vi "rad_Deploy Application Image.vi"(7 "App Image Temp Folder":path=path "C:/dev/Architectures/Reference Designs/Application Deployment and Replication/Application Deployment Utility/trunk/source/Application Images/_temp", 8 "error in (no error)":errorcluster, 10 "Selected Targets":T1[](array[typedef]) {"Primary NIC"."IP Address Request Mode" items=["Static"=1, "DHCP/Link-Local"=2, "Link-Local Only"=4, "DHCP Only"=8]}, 11 "App Image Path":path=path "C:/dev/Architectures/Reference Designs/Application Deployment and Replication/Application Deployment Utility/trunk/source/Application Images/AppImage1.lvappimg") -> (0 "error out":errorcluster, 1 "Cancelled":bool)   [LabVIEW 2021]
uses:
  Targets/TypeDefs/rad_Target Information.ctl
  Targets/TypeDefs/rad_Target Network Settings.ctl
  TypeDefs/rad_Target Configuration Settings.ctl
  TypeDefs/rad_Target Configuration Operations.ctl
  TypeDefs/rad_Deployment Notifiers.ctl
  TypeDefs/rad_Deployment Status Data Type.ctl
  TypeDefs/rad_Deployment Progress Data Type.ctl
  Util/FP Control/FP Control Functions.ctl
  <vilib>/Utility/error.llb/Clear Errors.vi
  NI-Auth/rad_IPaddr and Password Global.vi
  rad_Globals.vi
  <vilib>/nisyscfg/Initialize Session.vi
  <vilib>/nisyscfg/Close (System).vi
  NI-Auth/rad_Open Session.vi
  <vilib>/nisyscfg/nisyscfg.lvlib
panel:
  out "Stop Updates":bool
  in  "Deploy":bool
  in  "Config Options":bool
  in  "Log":bool
  in  "Stop":bool
  in  "State Variables":T6={"App Image Path"=path "C:/dev/Architectures/Reference Designs/Application Deployment and Replication/Application Deployment Utility/trunk/source/Application Images/AppImage1.lvappimg", "App Image Temp Folder"=path "C:/dev/Architectures/Reference Designs/Application Deployment and Replication/Application Deployment Utility/trunk/source/Application Images/_temp", "Targets"=[], "Target Configuration Options"={"NumInBatch"=0, "Target Config Operation"=enum."No Config", "Target Name"="", "Increment Static IPs"=FALSE, "Change Target Name"=FALSE, "Primary NIC"={"MAC address"="", "IP Address Request Mode"=2, "IP address"="", "Subnet mask"="", "Gateway"="", "DNS server"=""}}, "Deployment Notifiers"=[]} {"Target Configuration Options"."Primary NIC"."IP Address Request Mode" items=["Static"=1, "DHCP/Link-Local"=2, "Link-Local Only"=4, "DHCP Only"=8]; "Targets"."Primary NIC"."IP Address Request Mode" items=["Static"=1, "DHCP/Link-Local"=2, "Link-Local Only"=4, "DHCP Only"=8]}
  out "Targets":i32(listbox)
  in  "Close":bool
  # "Targets"
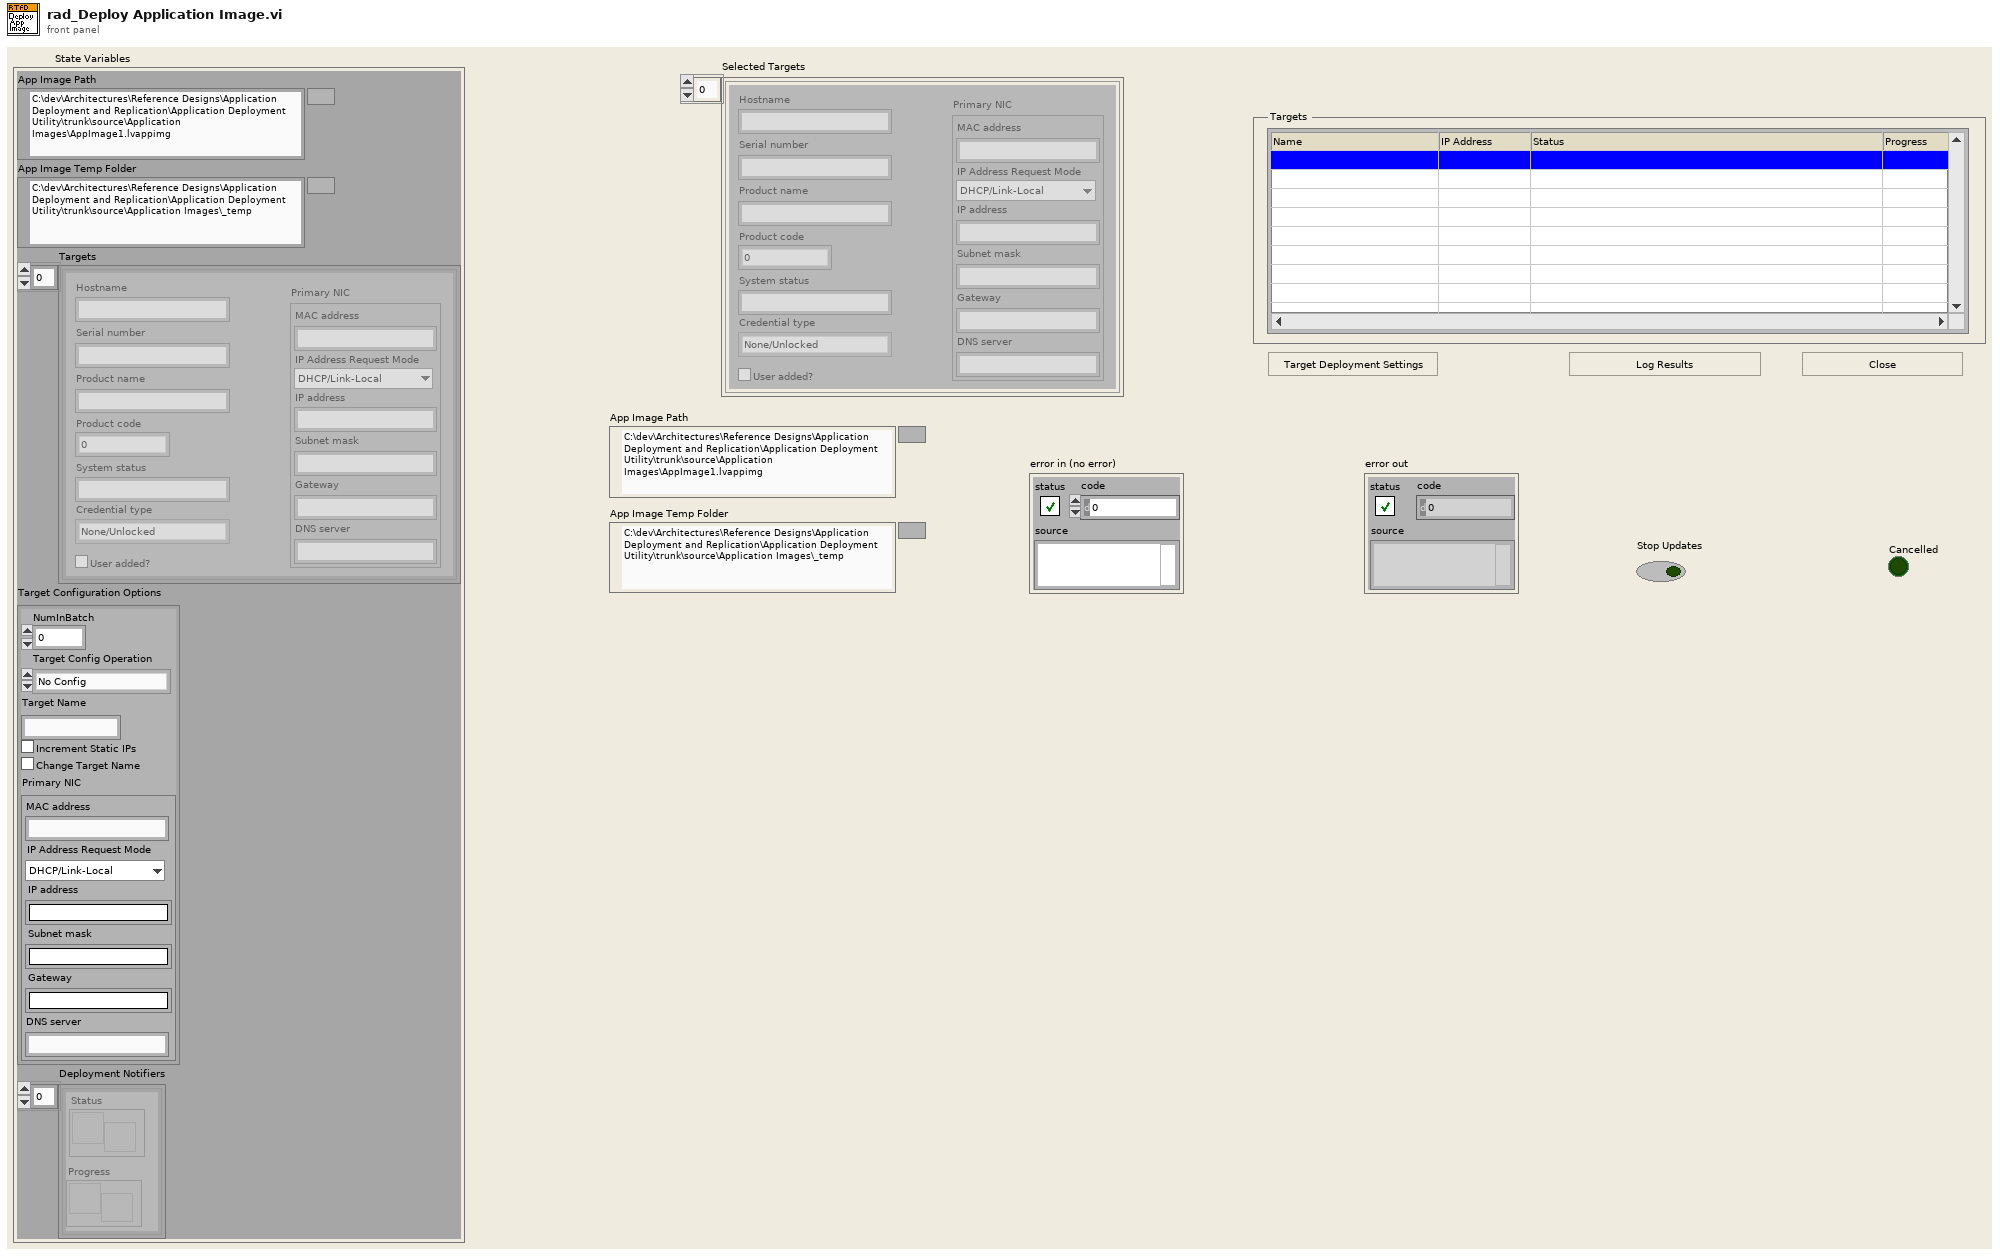
[diagram p1: front panel]
types:
  T1 = typedef "rad_Target Information.ctl" = cluster{"Hostname":string, "Serial number":string, "Product name":string, "Product code":i32, "System status":string, "Credential type":enum16{"None/Unlocked", "FTP Password", "NIAuth Credentials"}, "User added?":bool, "Primary NIC":T2}
  T2 = typedef "rad_Target Network Settings.ctl" = cluster{"MAC address":string, "IP Address Request Mode":i32, "IP address":string, "Subnet mask":string, "Gateway":string, "DNS server":string}
  T3 = typedef "rad_Target Configuration Settings.ctl" = cluster{"NumInBatch":u32, "Target Config Operation":T4, "Target Name":string, "Increment Static IPs":bool, "Change Target Name":bool, "Primary NIC":T2}
  T4 = typedef "rad_Target Configuration Operations.ctl" = enum8{"No Config", "Image Config", "Static Config"}
  T5 = typedef "rad_Deployment Notifiers.ctl" = cluster{"Status":refnum<notifier>, "Progress":refnum<notifier>}
  T6 = cluster{"App Image Path":path, "App Image Temp Folder":path, "Targets":T1[], "Target Configuration Options":T3, "Deployment Notifiers":T5[]}
  T7 = typedef "rad_Deployment Progress Data Type.ctl" = i8
  T8 = typedef "rad_Deployment Status Data Type.ctl" = string
  T9 = typedef "FP Control Functions.ctl" = enum16{"Open", "Close", "Bring To Front", "Center"}
  T10 = enum8{"Enabled", "Disabled", "Disabled and Grayed Out"}
  T11 = typedef "rad_Application Image Properties.ctl" = cluster{"Name":string, "Version":string, "Time":timestamp, "Description":string, "Key":string, "Chassis":string, "FPGA Properties":T12, "Model":string, "Retrieve":string[], "Deploy":string[], "Installed Software":string[]}
  T12 = typedef "rad_FPGA Properties.ctl" = T13[]
  T13 = typedef "rad_FPGA Flash Properties.ctl" = cluster{"Resource Name":string, "Path":path}
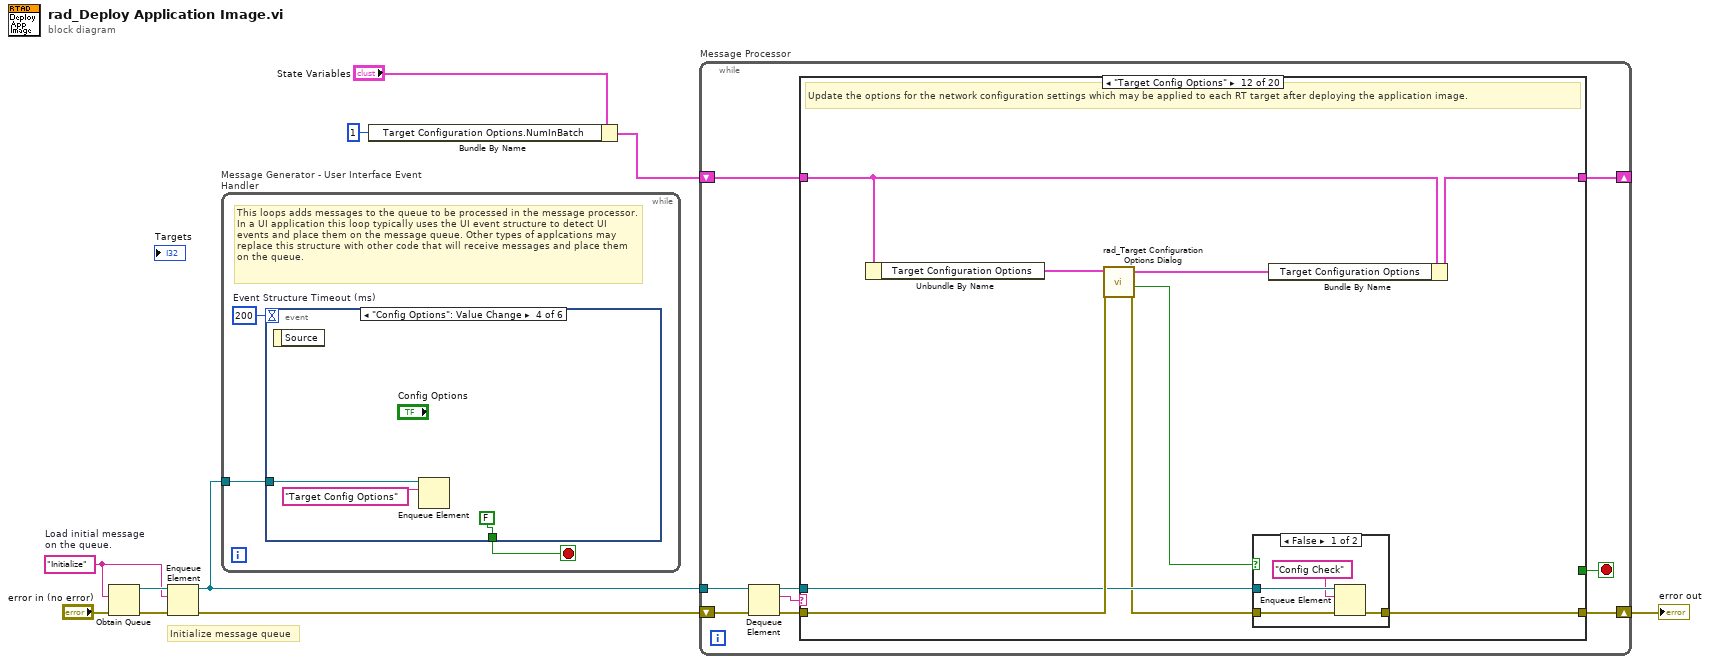
[diagram p0: block diagram]
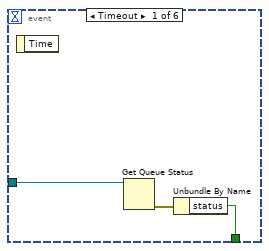
[diagram p2: hidden frame]
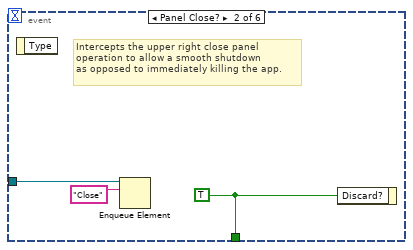
[diagram p3: hidden frame]
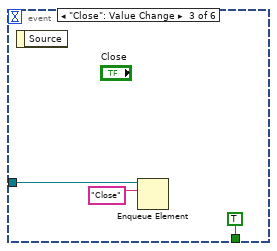
[diagram p4: hidden frame]
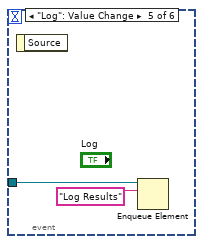
[diagram p5: hidden frame]
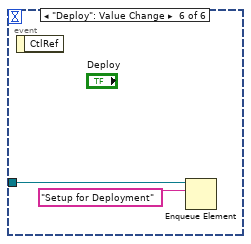
[diagram p6: hidden frame]
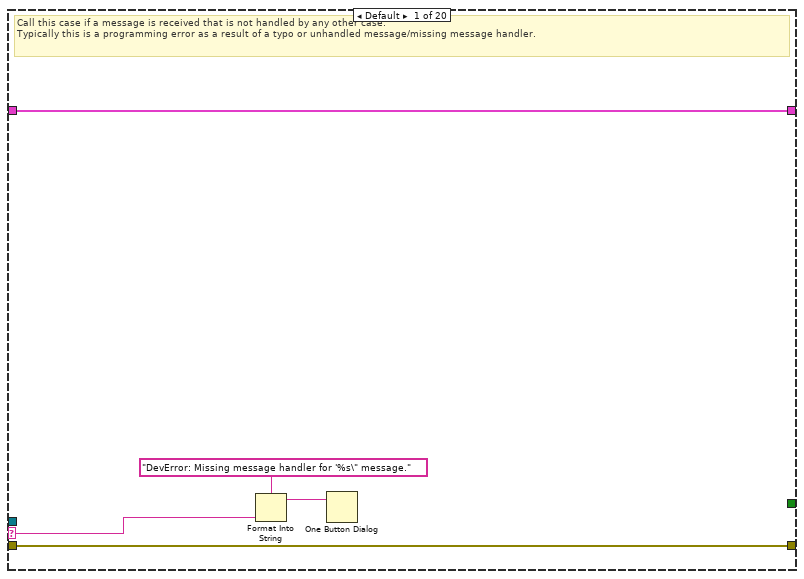
[diagram p7: hidden frame]
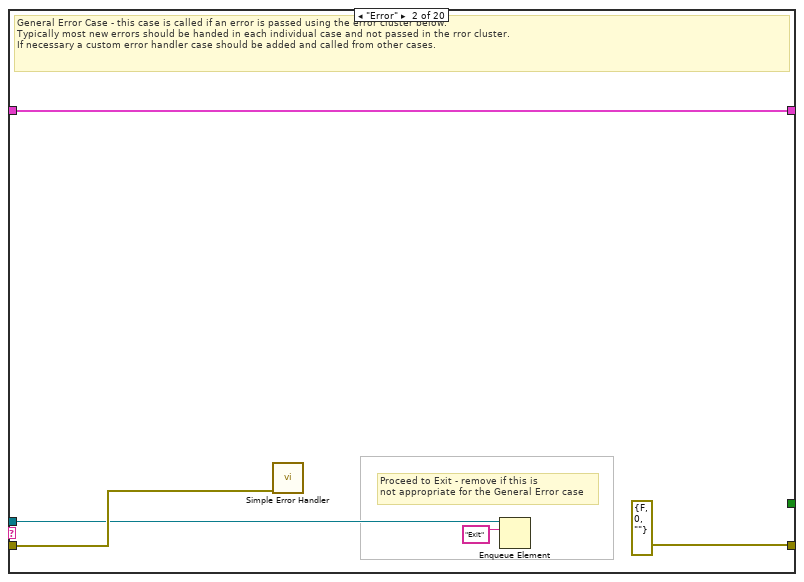
[diagram p8: hidden frame]
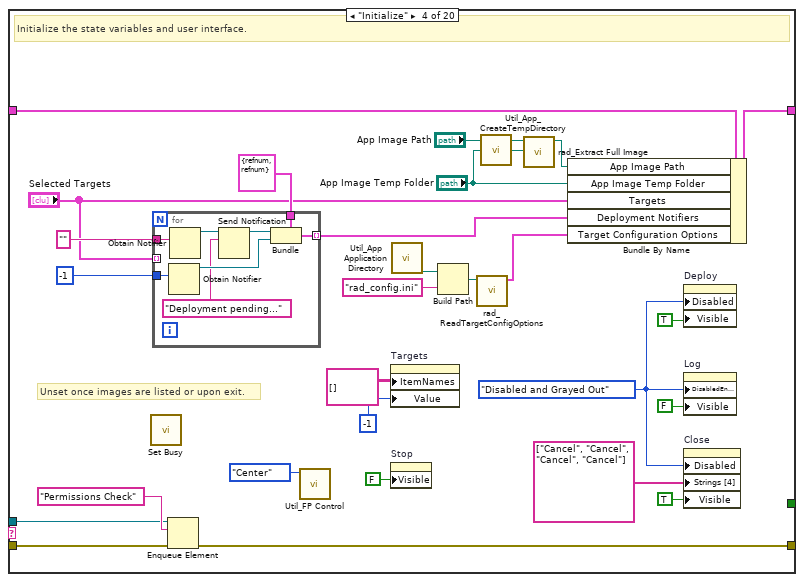
[diagram p10: hidden frame]
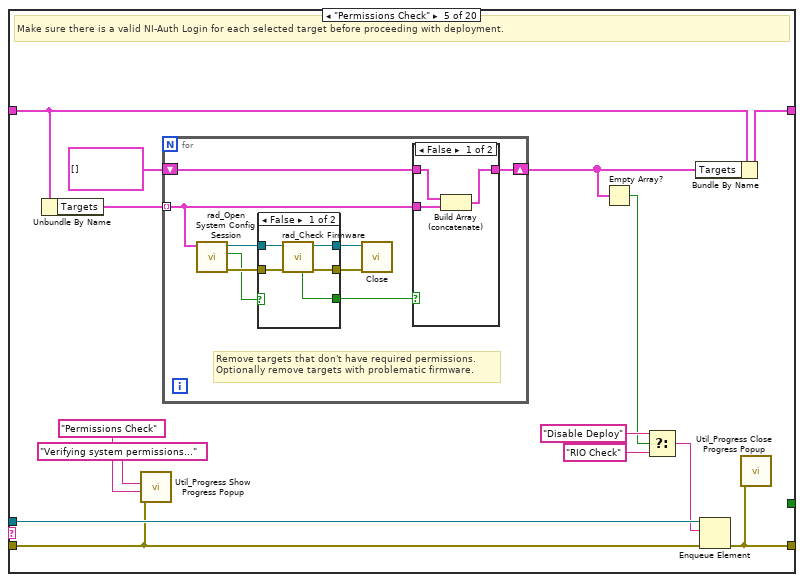
[diagram p11: hidden frame]
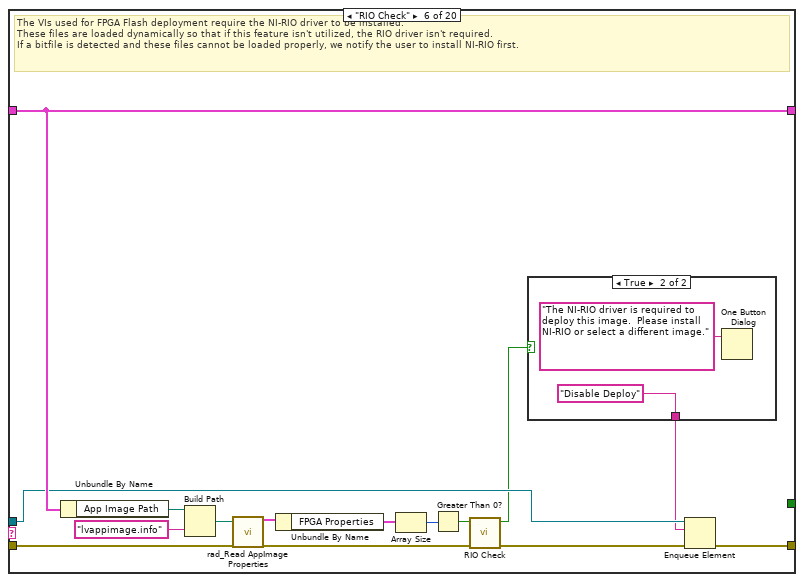
[diagram p14: hidden frame]
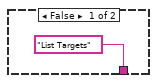
[diagram p15: hidden frame]
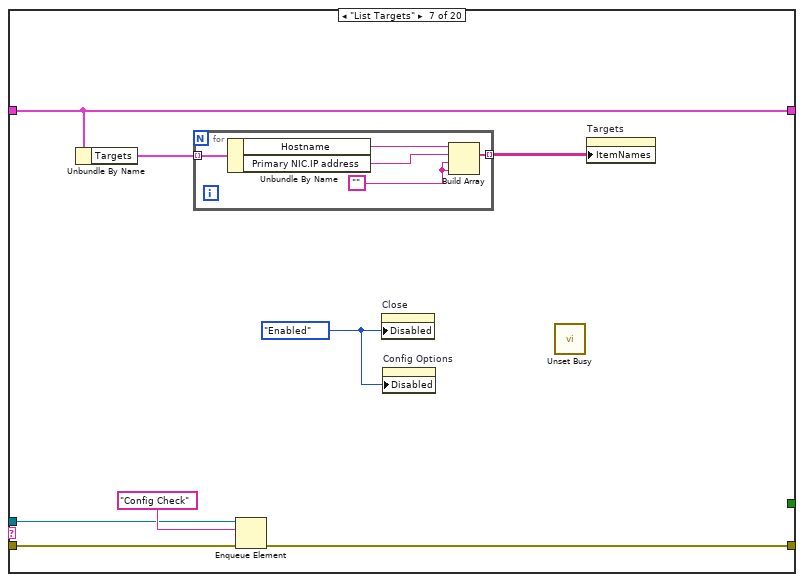
[diagram p16: hidden frame]
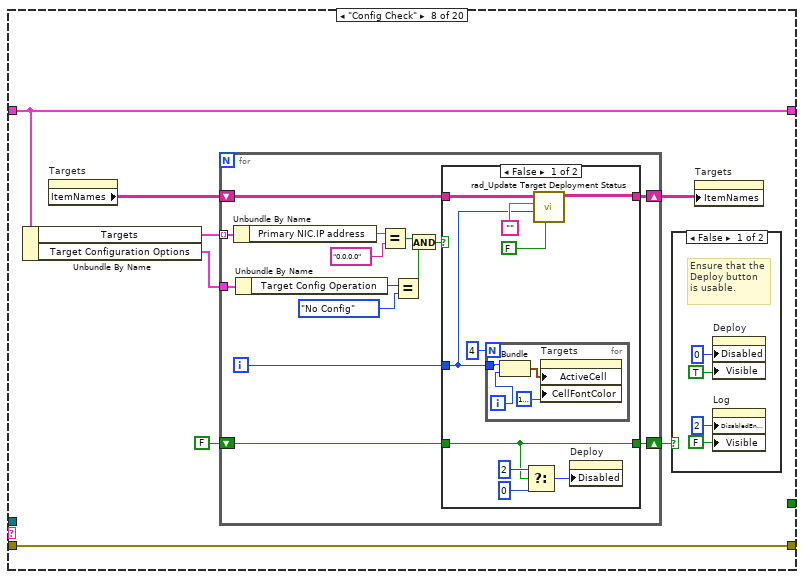
[diagram p17: hidden frame]
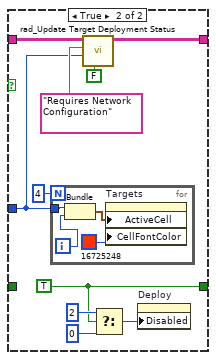
[diagram p19: hidden frame]
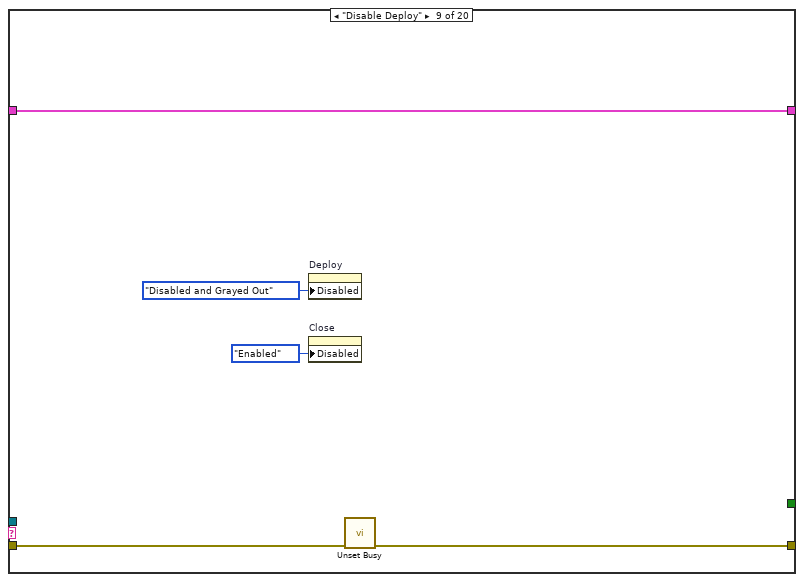
[diagram p20: hidden frame]
diagram:
  w4 = "Initialize"  # Load initial message on the queue.
  # "Initialize message queue"
  n1 = Obtain Queue(element data type=w4, error in (no error)="error in (no error)") -> (queue out=w6:refnum<queue>, error out=w10:errorcluster)  [unwired: 3 in, 1 out]
  n2 = Enqueue Element(queue=w6, element=w4, error in (no error)=w10) -> (queue out=w5:refnum<queue>, error out=w7:errorcluster)  [unwired: 1 in, 1 out]
  n3 = while "Message Generator - User Interface Event Handler" {
    tunnel: w5 -> [w11]
    stop <- w12 stop-if-true
    w13 = 200  # Event Structure Timeout (ms)
    # "This loops adds messages to the queue to be processed in the message processor. In a UI application this loop typically uses the UI event structure to detect UI events and place them on the message queue. Other types of applcations may replace this structure with other code that will receive messages and place them on the queue."
    n4 = event shown="[3] \"Config Options\": Value Change" {
      selector: _ -> [_ _ _ _ _ _]
      dyn-events: _ -> [_ _ _ _ _ _]
      timeout: w13 -> [_ _ _ _ _ _]
      tunnel: [w15 w19 TRUE ("Discard?") FALSE ("Discard?") _ _] -> w12
      tunnel: w11 -> [w14 w18 w22 w25 w27 w29]
      event Timeout {
        n5 = event-data() -> ()  [unwired: 2 out]
        n6 = Get Queue Status(queue=w14) -> (error out=w16:errorcluster)  [unwired: 2 in, 7 out]
        n7 = Unbundle By Name(w16) -> ("status"=w15:bool)
      }
      event Panel Close? {
        w19 = TRUE ("Discard?")
        # "Intercepts the upper right close panel\noperation to allow a smooth shutdown\nas opposed to immediately killing the app."
        n8 = event-data() -> ()  [unwired: 2 out]
        n9 = Enqueue Element(queue=w18, element="Close") -> ()  [unwired: 2 in, 3 out]
        n10 = event-data("Discard?"=w19) -> ()  [unwired: 1 in, 1 out]
      }
      event "Close": Value Change {
        n11 = event-data() -> ()  [unwired: 2 out]
        n12 = Enqueue Element(queue=w22, element="Close") -> ()  [unwired: 2 in, 3 out]
      }
      event "Config Options": Value Change {
        n13 = event-data() -> ()  [unwired: 2 out]
        n14 = Enqueue Element(queue=w25, element="Target Config Options") -> ()  [unwired: 2 in, 3 out]
      }
      event "Log": Value Change {
        n15 = event-data() -> ()  [unwired: 2 out]
        n16 = Enqueue Element(queue=w27, element="Log Results") -> ()  [unwired: 2 in, 3 out]
      }
      event "Deploy": Value Change {
        n17 = event-data() -> ()  [unwired: 2 out]
        n18 = Enqueue Element(queue=w29, element="Setup for Deployment") -> ()  [unwired: 2 in, 3 out]
      }
    }
  }
  n19 = Bundle By Name(cluster="State Variables", "Target Configuration Options.NumInBatch"=u32 1) -> (w2:T6)
  n20 = while "Message Processor" {
    shift-left: w7 -> [w33]
    shift-right: [w34] -> w8
    tunnel: w5 -> [w32]
    shift-left: w2 -> [w38]
    shift-right: [w37] -> _
    stop <- w30 stop-if-true
    n21 = Dequeue Element(queue=w32, error in (no error)=w33) -> (queue out=w36:refnum<queue>, element=w31:string, error out=w35:errorcluster)  [unwired: 1 in, 1 out]
    n22 = case shown="\"Target Config Options\"" w31 {
      selector: w31 -> [w41 _ _ _ _ _ _ _ _ _ _ _ _ _ _ _ _ _ _ _]
      tunnel: [w43 w48 w50 w77 w97 w133 w145 w155 w209 w213 w215 w221 w241 w260 w297 w305 w307 w315 w318 w325] -> w37
      tunnel: w38 -> [w43 w48 w50 w78 w98 w133 w145 w155 w209 w213 w215 w222 w241 w260 w297 w305 w307 w315 w318 w325]
      tunnel: w36 -> [_ w45 _ w56 w96 w130 w140 _ _ _ _ w219 w237 w255 _ _ _ w309 _ w330]
      tunnel: w35 -> [w42 w46 w49 w72 w92 w125 w142 w160 w211 w212 w214 w223 w242 w259 w298 w303 w306 w310 w316 w331]
      tunnel: [w42 errorcluster {"status"=FALSE, "code"=0, "source"=""} ("error out") w49 w58 w91 w131 w141 w160 w210 w212 w214 w217 w233 w253 w298 w302 w306 w308 w316 w322] -> w34
      tunnel: [_ _ _ _ _ _ _ _ _ _ _ _ _ _ _ _ _ _ _ TRUE] -> w30
      frame Default {
        # "Call this case if a message is received that is not handled by any other case.\nTypically this is a programming error as a result of a typo or unhandled message/missing message handler."
        n23 = Format Into String(format string="DevError: Missing message handler for '%s\" message." ("message"), w41) -> (resulting string=w39:string)  [unwired: 2 in, 1 out]
        n24 = One Button Dialog(message=w39) -> ()  [unwired: 2 out]
      }
      frame "Error" {
        # "Proceed to Exit - remove if this is\nnot appropriate for the General Error case"
        # "General Error Case - this case is called if an error is passed using the error cluster below.\nTypically most new errors should be handed in each individual case and not passed in the rror cluster.\nIf necessary a custom error handler case should be added and called from other cases."
        n25 = call <vilib>:"Simple Error Handler.vi"("error in (no error)"=w46) -> ()  [unwired: 1 in, 8 out]
        n26 = Enqueue Element(queue=w45, element="Exit") -> ()  [unwired: 2 in, 3 out]
      }
      frame "*******Init******" {
        # "Dummy case to add a seperator in the Case Structure menu."
      }
      frame "Initialize" {
        w51 = T10."Disabled and Grayed Out" ("Disabled")
        # "Unset once images are listed or upon exit."
        # "Initialize the state variables and user interface."
        n27 = call <vilib>:"Set Busy.vi"() -> ()  [unwired: 10 in, 2 out]
        n28 = for {
          tunnel: T8 "" ("status notifier data type") -> [w86]
          tunnel: T7 -1 ("Progress") -> [w85]
          tunnel: T5 {"Status"=refnum, "Progress"=refnum} ("Deployment Notifiers") -> [w83]
          tunnel: [w82] -> w67 mode=indexing
          tunnel: "Selected Targets" -> [_] mode=indexing
          n29 = Obtain Notifier(notification data type=w85) -> (notifier out=w84:refnum<notifier>)  [unwired: 3 in, 2 out]
          n30 = Obtain Notifier(notification data type=w86) -> (notifier out=w81:refnum<notifier>)  [unwired: 3 in, 2 out]
          n31 = Send Notification(notification=T8 "Deployment pending...", notifier=w81) -> (notifier out=w80:refnum<notifier>)  [unwired: 1 in, 1 out]
          n32 = Bundle(cluster=w83, "Status"=w80, "Progress"=w84) -> (w82:T5)
        }
        n33 = Enqueue Element(queue=w56, element="Permissions Check", error in (no error)=w72) -> (error out=w58:errorcluster)  [unwired: 1 in, 2 out]
        n34 = call "Util_FP Control.vi"("Function"=FP_Control_Functions."Center") -> ()  [unwired: 1 in, 10 out]
        n35 = property on="Targets" class="MCListbox (strict)"("ItemNames"=string[][] [] ("Item Names"), "Value"=-1 ("Targets")) -> ()  [unwired: 2 in, 2 out]
        n36 = property on="Stop" class="Bool"("Visible"=FALSE) -> ()  [unwired: 2 in, 2 out]
        n37 = call "Util_App Application Directory.vi"() -> ("Application Directory"=w66:path)  [unwired: 11 out]
        n38 = Build Path(base path=w66, name or relative path="rad_config.ini" ("Config File Name")) -> (appended path=w64:path)
        n39 = call "rad_ReadTargetConfigOptions.vi"("configuration file path"=w64) -> ("TargetConfigurationOptions"=w63:T3)  [unwired: 9 in, 1 out]
        n40 = call "Util_App_CreateTempDirectory.vi"("TempFolderPath"="App Image Temp Folder") -> ("TempFolderPath_out"=w60:path)
        n41 = call "rad_Extract Full Image.vi"("App Image Temp Folder"=w60, "Zipped App Image File Path"="App Image Path") -> ("Unzipped App Image Folder Path"=w61:path)  [unwired: 8 in, 1 out]
        n42 = Bundle By Name(cluster=w78, "App Image Path"=w61, "App Image Temp Folder"="App Image Temp Folder", "Targets"="Selected Targets", "Deployment Notifiers"=w67, "Target Configuration Options"=w63) -> (w77:T6)
        n43 = property on="Deploy" class="Bool"("Disabled"=w51, "Visible"=TRUE) -> ()  [unwired: 2 in, 2 out]
        n44 = property on="Log" class="Bool"("DisabledEnum"=w51, "Visible"=FALSE) -> ()  [unwired: 2 in, 2 out]
        n45 = property on="Close" class="Bool"("Disabled"=w51, "Strings [4]"=string[] ["Cancel", "Cancel", "Cancel", "Cancel"], "Visible"=TRUE) -> ()  [unwired: 2 in, 2 out]
      }
      frame "Permissions Check" {
        # "Make sure there is a valid NI-Auth Login for each selected target before proceeding with deployment."
        n46 = Unbundle By Name(w98) -> ("Targets"=w100:T1[])
        n47 = call "Util_Progress Show Progress Popup.vi"("error in (no error)"=w92, "Title"="Permissions Check" ("Message"), "Message"="Verifying system permissions...") -> ()  [unwired: 8 in, 1 out]
        n48 = for {
          tunnel: w100 -> [w107] mode=indexing
          shift-right: [w109] -> w88
          shift-left: T1[] [] -> [w108]
          # "Remove targets that don't have required permissions.\nOptionally remove targets with problematic firmware."
          n49 = call "rad_Open System Config Session.vi"("Target settings"=w107) -> ("error out"=w106:errorcluster, "Cancelled"=w101:bool, "Session out"=w104:refnum<k21>)  [unwired: 7 in, 1 out]
          n50 = case shown="False" w101 {
            selector: w101 -> [_ w115]
            tunnel: w106 -> [w114 w117]
            tunnel: [w111 w117] -> w105
            tunnel: w104 -> [w113 w116]
            tunnel: [w112 w116] -> w103
            tunnel: [w110 w115] -> w102
            frame False {
              n51 = call "rad_Check Firmware.vi"("error in (no error)"=w114, "System Configuration"=w113) -> ("error out"=w111:errorcluster, "System Configuration out"=w112:refnum<k21>, "Bad firmware and user canceled"=w110:bool)  [unwired: 7 in]
            }
            frame True {
            }
          }
          n52 = call-poly <vilib>:"Close.vi"("error in (no error)"=w105, "Session in"=w103) -> ()  [unwired: 9 in, 1 out]
          n53 = case shown="False" w102 {
            tunnel: w107 -> [w120 _]
            tunnel: [w119 w121] -> w109
            tunnel: w108 -> [w118 w121]
            frame False {
              n54 = Build Array (concatenate)(w118, w120) -> (w119:T1[])
            }
            frame True {
            }
          }
        }
        n55 = Empty Array?(array=w88) -> (empty?=w87:bool)
        n56 = Select(t="Disable Deploy", s=w87, f="RIO Check") -> (s? t:f=w93:string)
        n57 = Bundle By Name(cluster=w98, "Targets"=w88) -> (w97:T6)
        n58 = Enqueue Element(queue=w96, element=w93, error in (no error)=w92) -> (error out=w91:errorcluster)  [unwired: 1 in, 2 out]
        n59 = call "Util_Progress Close Progress Popup.vi"("error in (no error)"=w91) -> ()  [unwired: 10 in, 1 out]
      }
      frame "RIO Check" {
        # "The VIs used for FPGA Flash deployment require the NI-RIO driver to be installed.  \nThese files are loaded dynamically so that if this feature isn't utilized, the RIO driver isn't required.\nIf a bitfile is detected and these files cannot be loaded properly, we notify the user to install NI-RIO first."
        n60 = Unbundle By Name(w133) -> ("App Image Path"=w123:path)
        n61 = Build Path(base path=w123, name or relative path="lvappimage.info") -> (appended path=w122:path)
        n62 = call "rad_Read AppImage Properties.vi"("AppImage Properties Path"=w122, "error in (no error)"=w125) -> ("AppImage Properties"=w126:T11, "error out"=w127:errorcluster)  [unwired: 12 in, 4 out]
        n63 = Unbundle By Name(w126) -> ("FPGA Properties"=w136:T12)
        n64 = Array Size(array=w136) -> (size(s)=w135:i32)
        n65 = Greater Than 0?(x=w135) -> (x > 0?=w134:bool)
        n66 = call "RIO Check.vi"("error in"=w127, "Requires RIO"=w134) -> ("error out"=w132:errorcluster, "RIO needed but not installed"=w129:bool)  [unwired: 8 in]
        n67 = case shown="True" w129 {
          tunnel: ["List Targets" "Disable Deploy" ("t")] -> w128
          frame False {
          }
          frame True {
            n68 = One Button Dialog(message="The NI-RIO driver is required to deploy this image.  Please install NI-RIO or select a different image.") -> ()  [unwired: 1 in, 1 out]
          }
        }
        n69 = Enqueue Element(queue=w130, element=w128, error in (no error)=w132) -> (error out=w131:errorcluster)  [unwired: 1 in, 2 out]
      }
      frame "List Targets" {
        w144 = T10."Enabled" ("Disabled")
        n70 = Unbundle By Name(w145) -> ("Targets"=w147:T1[])
        n71 = for {
          tunnel: w147 -> [w152] mode=indexing
          tunnel: [w149] -> w146 mode=indexing
          w148 = ""
          n72 = Unbundle By Name(w152) -> ("Hostname"=w151:string, "Primary NIC.IP address"=w150:string)
          n73 = Build Array(w151, w150, w148, w148) -> (w149:string[])
        }
        n74 = Enqueue Element(queue=w140, element="Config Check", error in (no error)=w142) -> (error out=w141:errorcluster)  [unwired: 1 in, 2 out]
        n75 = property on="Close" class="Bool"("Disabled"=w144) -> ()  [unwired: 2 in, 2 out]
        n76 = property on="Config Options" class="Bool"("Disabled"=w144) -> ()  [unwired: 2 in, 2 out]
        n77 = call <vilib>:"Unset Busy.vi"() -> ()  [unwired: 11 in, 1 out]
        n78 = property on="Targets" class="MCListbox (strict)"("ItemNames"=w146) -> ()  [unwired: 2 in, 2 out]
      }
      frame "Config Check" {
        n79 = Unbundle By Name(w155) -> ("Targets"=w158:T1[], "Target Configuration Options"=w159:T3)
        n80 = property on="Targets" class="MCListbox (strict)"() -> ("ItemNames"=w154:string[][])  [unwired: 2 in, 2 out]
        n81 = for {
          tunnel: w158 -> [w169] mode=indexing
          tunnel: w159 -> [w168]
          shift-right: [w165] -> w153
          shift-left: FALSE -> [w166]
          shift-right: [w171] -> w156
          shift-left: w154 -> [w167]
          i -> [w170]
          n82 = Unbundle By Name(w169) -> ("Primary NIC.IP address"=w178:string)
          n83 = Unbundle By Name(w168) -> ("Target Config Operation"=w176:T4)
          n84 = Equal?(x=w178, y="0.0.0.0") -> (x = y?=w174:bool)
          n85 = Equal?(x=w176, y=rad_Target_Configuration_Operations."No Config") -> (x = y?=w172:bool)
          n86 = And(x=w174, y=w172) -> (x .and. y?=w173:bool)
          n87 = case shown="False" w173 {
            tunnel: [w187 w202] -> w171
            tunnel: w170 -> [w185 w198]
            tunnel: w167 -> [w188 w199]
            tunnel: w166 -> [w180 _]
            tunnel: [w180 w195] -> w165
            frame False {
              n88 = for {
                N: 4 -> [_]
                tunnel: w185 -> [w191]
                i -> [w190]
                n89 = Bundle(w191, w190) -> (w189:cluster{i32, i32})  [unwired: 1 in]
                n90 = property on="Targets" class="MCListbox (strict)"("ActiveCell"=w189, "CellFontColor"=u32 16777222) -> ()  [unwired: 2 in, 2 out]
              }
              n91 = Select(t=2, s=w180, f=0) -> (s? t:f=w181:i32)
              n92 = call "rad_Update Target Deployment Status.vi"("Add Timestamp?"=FALSE, "Target Index"=w185, "Message"="", "Targets Deployment Status"=w188) -> ("Targets Deployment Status"=w187:string[][])  [unwired: 7 in]
              n93 = property on="Deploy" class="Bool"("Disabled"=w181) -> ()  [unwired: 2 in, 2 out]
            }
            frame True {
              w195 = TRUE
              n94 = for {
                N: 4 -> [_]
                tunnel: w198 -> [w205]
                i -> [w204]
                n95 = Bundle(w205, w204) -> (w203:cluster{i32, i32})  [unwired: 1 in]
                n96 = property on="Targets" class="MCListbox (strict)"("ActiveCell"=w203, "CellFontColor"=u32 16725248) -> ()  [unwired: 2 in, 2 out]
              }
              n97 = call "rad_Update Target Deployment Status.vi"("Add Timestamp?"=FALSE, "Target Index"=w198, "Message"="Requires Network Configuration", "Targets Deployment Status"=w199) -> ("Targets Deployment Status"=w202:string[][])  [unwired: 7 in]
              n98 = Select(t=2, s=w195, f=0) -> (s? t:f=w194:i32)
              n99 = property on="Deploy" class="Bool"("Disabled"=w194) -> ()  [unwired: 2 in, 2 out]
            }
          }
        }
        n100 = case shown="False" w153 {
          frame False {
            # "Ensure that the\nDeploy button\nis usable."
            n101 = property on="Deploy" class="Bool"("Disabled"=0, "Visible"=TRUE) -> ()  [unwired: 2 in, 2 out]
            n102 = property on="Log" class="Bool"("DisabledEnum"=2, "Visible"=FALSE) -> ()  [unwired: 2 in, 2 out]
          }
          frame True {
          }
        }
        n103 = property on="Targets" class="MCListbox (strict)"("ItemNames"=w156) -> ()  [unwired: 2 in, 2 out]
      }
      frame "Disable Deploy" {
        n104 = property on="Deploy" class="Bool"("Disabled"=T10."Disabled and Grayed Out") -> ()  [unwired: 2 in, 2 out]
        n105 = property on="Close" class="Bool"("Disabled"=T10."Enabled") -> ()  [unwired: 2 in, 2 out]
        n106 = call <vilib>:"Unset Busy.vi"("error in (no error)"=w211) -> ("error out"=w210:errorcluster)  [unwired: 10 in]
      }
      frame "*****************" {
        # "Dummy case to add a seperator in the Case Structure menu."
      }
      frame "Update Display" {
      }
      frame "Target Config Options" {
        # "Update the options for the network configuration settings which may be applied to each RT target after deploying the application image."
        n107 = Unbundle By Name(w222) -> ("Target Configuration Options"=w224:T3)
        n108 = call "rad_Target Configuration Options Dialog.vi"("error in"=w223, "Target Configuration Options"=w224) -> ("error out"=w218:errorcluster, "Cancelled"=w216:bool, "Target Configuration Options"=w220:T3)  [unwired: 7 in]
        n109 = case shown="False" w216 {
          tunnel: w219 -> [w228 _]
          tunnel: w218 -> [w227 w229]
          tunnel: [w226 w229] -> w217
          frame False {
            n110 = Enqueue Element(queue=w228, element="Config Check" ("Message Name"), error in (no error)=w227) -> (error out=w226:errorcluster)  [unwired: 1 in, 2 out]
          }
          frame True {
          }
        }
        n111 = Bundle By Name(cluster=w222, "Target Configuration Options"=w220) -> (w221:T6)
      }
      frame "Setup for Deployment" {
        w239 = T10."Disabled and Grayed Out" ("Disabled")
        # "Update the UI for the deployment process - disable some buttons."
        n112 = Enqueue Element(queue=w237, element="Deploy Application Image", error in (no error)=w242) -> (queue out=w234:refnum<queue>, error out=w235:errorcluster)  [unwired: 1 in, 1 out]
        n113 = property on="Stop" class="Bool"("Visible"=TRUE) -> ()  [unwired: 2 in, 2 out]
        n114 = property on="Close" class="Bool"("Disabled"=w239, "Visible"=FALSE) -> ()  [unwired: 2 in, 2 out]
        n115 = property on="Config Options" class="Bool"("Disabled"=w239) -> ()  [unwired: 2 in, 2 out]
        n116 = property on="Log" class="Bool"("Disabled"=w239, "Visible"=TRUE) -> ()  [unwired: 2 in, 2 out]
        n117 = Enqueue Element(queue=w234, element="Cleanup from Deployment", error in (no error)=w235) -> (error out=w233:errorcluster)  [unwired: 1 in, 2 out]
        n118 = property on="Deploy" class="Bool"("Visible"=FALSE) -> ()  [unwired: 2 in, 2 out]
      }
      frame "Deploy Application Image" {
        # "Deploy the specified image to the selected targets in parallel, in batches up to the Deployment Batch Size.\nIf an error occurs, display it for the relevant target, but don't pass it out the error wire.\nThis allows deployment to succeed for as many targets as possible."
        n119 = Unbundle By Name(w260) -> ("Deployment Notifiers"=w250:T5[], "App Image Temp Folder"=w261:path, "App Image Path"=w263:path, "Targets"=w262:T1[], "Target Configuration Options"=w244:T3)
        n120 = control-ref of="Targets"() -> (w251:refnum<vi>)
        n121 = control-ref of="Stop Updates"() -> (w246:refnum<vi>)
        n122 = Unbundle By Name(w244) -> ("NumInBatch"=w243:u32)
        n123 = Array Size(array=w250) -> (size(s)=w258:i32)
        n124 = Divide(x=w258, y=w243) -> (x/y=w257:dbl)
        n125 = Round Toward +Infinity(x=w257) -> (ceil(x): smallest int >= x=w256:dbl)
        n126 = for {
          N: w256 -> [_]
          tunnel: w263 -> [w290]
          tunnel: w262 -> [w285]
          tunnel: w261 -> [w289]
          tunnel: w243 -> [w282]
          shift-right: [w281] -> w254
          shift-left: w259 -> [w288]
          tunnel: [w279] -> w252
          tunnel: w250 -> [w278]
          tunnel: [TRUE] -> w249
          shift-right: [w276] -> _
          shift-left: w244 -> [w291]
          i -> [w287]
          stop <- w279 stop-if-true
          n127 = Multiply(x=w282, y=w287) -> (x*y=w283:u32)
          n128 = Array Subset(array=w285, index=w283, length=w282) -> (w284:T1[])
          n129 = Array Subset(array=w278, index=w283, length=w282) -> (w286:T5[])
          n130 = call "rad_Deploy Images with Progress.vi"("Deployment Notifiers"=w286, "temp folder"=w289, "error in (no error)"=w288, "Target Config Options in"=w291, "RT Deployment Targets in"=w284, "image path"=w290) -> ("error out"=w280:errorcluster, "Target Config Options out"=w276:T3)  [unwired: 3 in, 1 out]
          n131 = flat-sequence {
            tunnel: ["Stop"] -> w279
            tunnel: [w292] -> w281
            tunnel: w280 -> [w292]
            frame #0 {
            }
          }
        }
        n132 = flat-sequence {
          tunnel: w250 -> [w266]
          tunnel: w251 -> [w267]
          tunnel: [w267] -> w248
          tunnel: [w266] -> w247
          tunnel: w246 -> [w265]
          tunnel: [w265] -> w245
          tunnel: w248 -> [w270]
          tunnel: w247 -> [w269]
          tunnel: w245 -> [w268]
          frame #0 {
            "Stop Updates" <- FALSE ("Stop Updates")
          }
          frame #1 {
            n133 = call "rad_Update Display.vi"("Deployment Notifiers"=w269, "Stop Updates"=w268, "Listbox Reference"=w270) -> ()  [unwired: 9 in]
          }
        }
        n134 = local write "Stop Updates"(w249) -> ()
        n135 = case shown="True" w252 {
          tunnel: w255 -> [_ w275]
          tunnel: w254 -> [w271 w274]
          tunnel: [w271 w273] -> w253
          frame False {
          }
          frame True {
            n136 = Enqueue Element(queue=w275, element="Close" ("Message Name"), error in (no error)=w274) -> (error out=w273:errorcluster)  [unwired: 1 in, 2 out]
          }
        }
      }
      frame "Cleanup from Deployment" {
        w295 = T10."Enabled" ("Disabled")
        # "Reset the UI after the deployment process."
        n137 = property on="Config Options" class="Bool"("Disabled"=w295) -> ()  [unwired: 2 in, 2 out]
        n138 = property on="Log" class="Bool"("Disabled"=w295) -> ()  [unwired: 2 in, 2 out]
        n139 = property on="Close" class="Bool"("Disabled"=w295, "Strings [4]"=string[] ["Close", "Close", "Close", "Close"], "Visible"=TRUE) -> ()  [unwired: 2 in, 2 out]
        n140 = property on="Stop" class="Bool"("Visible"=FALSE) -> ()  [unwired: 2 in, 2 out]
      }
      frame "Log Results" {
        # "Log the deployment information and results to a TSV file."
        n141 = Unbundle By Name(w305) -> ("Targets"=w304:T1[], "App Image Path"=w301:path)
        n142 = property on="Targets" class="MCListbox (strict)"() -> ("ItemNames"=w300:string[][])  [unwired: 2 in, 2 out]
        n143 = call "rad_Write Deployment Results to File.vi"("error in"=w303, "App Image Path"=w301, "Targets Deployment"=w300, "Targets"=w304) -> ("error out"=w302:errorcluster)  [unwired: 1 in, 6 out]
      }
      frame "******Close******" {
        # "Dummy case to add a seperator in the Case Structure menu."
      }
      frame "Close" {
        n144 = Enqueue Element(queue=w309, element="Cleanup Temp App Image", error in (no error)=w310) -> (queue out=w312:refnum<queue>, error out=w313:errorcluster)  [unwired: 1 in, 1 out]
        n145 = Enqueue Element(queue=w312, element="Exit", error in (no error)=w313) -> (error out=w308:errorcluster)  [unwired: 1 in, 2 out]
      }
      frame "Cleanup Temp App Image" {
        # "Empty the temp folder used during deployment."
        n146 = Unbundle By Name(w318) -> ("App Image Temp Folder"=w317:path)
        n147 = Delete(path (use dialog)=w317, entire hierarchy (F)=TRUE) -> ()  [unwired: 1 in, 5 out]
      }
      frame "Exit" {
        n148 = Unbundle By Name(w325) -> ("Deployment Notifiers"=w324:T5[])
        n149 = Release Queue(queue=w330, force destroy? (F)=TRUE, error in (no error)=w331) -> (error out=w323:errorcluster)  [unwired: 2 out]
        n150 = for {
          tunnel: w324 -> [w337] mode=indexing
          shift-right: [w332] -> w322
          shift-left: w323 -> [w335]
          n151 = Unbundle By Name(w337) -> ("Status"=w336:refnum<notifier>, "Progress"=w334:refnum<notifier>)
          n152 = Release Notifier(notifier=w336, force destroy? (F)=TRUE, error in (no error)=w335) -> (error out=w333:errorcluster)  [unwired: 2 out]
          n153 = Release Notifier(notifier=w334, force destroy? (F)=TRUE, error in (no error)=w333) -> (error out=w332:errorcluster)  [unwired: 2 out]
        }
        n154 = property on="Close" class="Bool"() -> ("Strings [4]"=w329:string[])  [unwired: 2 in, 2 out]
        n155 = Index Array(array=w329) -> (element=w328:string)  [unwired: 1 in]
        n156 = Equal?(x="Cancel", y=w328) -> (x = y?=→"Cancelled":bool)
        n157 = call <vilib>:"Unset Busy.vi"() -> ()  [unwired: 11 in, 1 out]
      }
    }
  }
  "error out" <- w8
